vi "Gamma jj' Magnitude.vi"(1 "n'":i32, 2 "m,m' != 0":bool, 3 "n":i32) -> (0 "Magnitude":dbl)   [LabVIEW 2013, in "Zernike Polynome.lvlib"]
doc: "This VI calculates the magnitude of gamma jj'."
uses:
  Zernike Polynome.lvlib
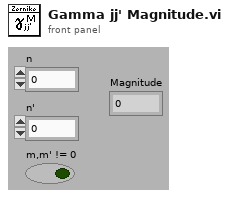
[diagram p1: front panel]
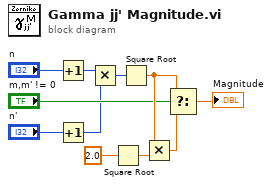
[diagram p0: block diagram]
diagram:
  n1 = Increment(x="n") -> (x+1=w4:i32)
  n2 = Increment(x="n'") -> (x+1=w3:i32)
  n3 = Multiply(x=w4, y=w3) -> (x*y=w5:i32)
  n4 = Square Root(x=2.0) -> (sqrt(x)=w7:dbl)
  n5 = Square Root(x=w5) -> (sqrt(x)=w10:dbl)
  n6 = Multiply(x=w10, y=w7) -> (x*y=w8:dbl)
  n7 = Select(t=w10, s="m,m' != 0", f=w8) -> (s? t:f=→"Magnitude":dbl)
